vi "pcfs_next_state.vi"(4 "total_steps":u32, 6 "current_iteration":u32, 7 "next_state":T1, 8 "error in (no error)":errorcluster, 11 "pcfs in":refnum<class "pcfs.lvclass">) -> (0 "error out":errorcluster, 1 "end_experiment":bool, 3 "pcfs out":refnum<class "pcfs.lvclass">, 5 "finish_position":bool)   [LabVIEW 2015, in "pcfs.lvclass"]
uses:
  pcfs.lvclass
  spcfs_fsm_tasks.ctl
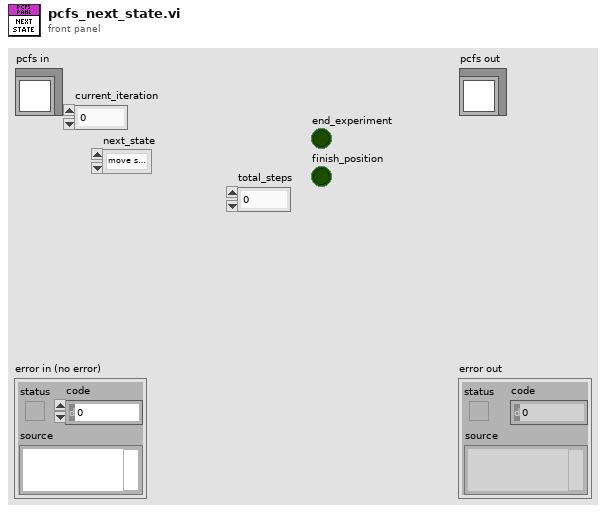
[diagram p1: front panel]
types:
  T1 = typedef "spcfs_fsm_tasks.ctl" = enum16{"move stage, start dither", "collect stream", "stop dither", "finish_position"}
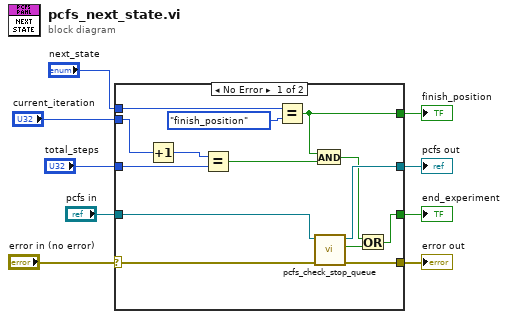
[diagram p0: block diagram]
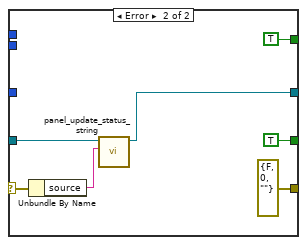
[diagram p2: hidden frame]
diagram:
  n1 = case shown="No Error" "error in (no error)" {
    selector: "error in (no error)" -> [w19 w27]
    tunnel: [w22 errorcluster {"status"=FALSE, "code"=0, "source"=""} ("error out")] -> w8
    tunnel: [w23 w28] -> w6
    tunnel: "pcfs in" -> [w20 w29]
    tunnel: "current_iteration" -> [w18 _]
    tunnel: "total_steps" -> [w21 _]
    tunnel: [w15 TRUE] -> w3
    tunnel: "next_state" -> [w14 _]
    tunnel: [w12 TRUE] -> w1
    frame No Error {
      n2 = Increment(x=w18) -> (x+1=w17:u32)
      n3 = Equal?(x=w17, y=w21) -> (x = y?=w11:bool)
      n4 = Equal?(x=w14, y=spcfs_fsm_tasks."finish_position") -> (x = y?=w12:bool)
      n5 = And(x=w12, y=w11) -> (x .and. y?=w10:bool)
      n6 = call "pcfs_check_stop_queue.vi"("error in (no error)"=w19, "scan_panel in"=w20) -> ("error out"=w22:errorcluster, "stop?"=w16:bool, "scan_panel out"=w23:refnum<class "pcfs.lvclass">)  [unwired: 7 in]
      n7 = Or(x=w10, y=w16) -> (x .or. y?=w15:bool)
    }
    frame Error {
      n8 = Unbundle By Name(w27) -> ("source"=w26:string)
      n9 = call-dynamic "panel_update_status_string.vi"("String"=w26, "scan_panel in"=w29) -> ("scan_panel out"=w28:refnum<class "pcfs.lvclass">)  [unwired: 8 in, 1 out]
    }
  }
  "error out" <- w8
  "pcfs out" <- w6
  "end_experiment" <- w3
  "finish_position" <- w1
